vi "Quaternion Between Vectors.vi"(9 "b":dbl[](array[numeric]), 11 "a":dbl[](array[numeric])) -> (3 "quaternion":T1)   [LabVIEW 2013]
uses:
  <vilib>/robotics/Kinematics/Quaternion.ctl
  <vilib>/Analysis/_algsub.llb/Real Vector Norm.vi
  <vilib>/Analysis/baseanly.llb/Real Dot Product.vi
  <vilib>/Analysis/NI_AALPro.lvlib
  <vilib>/Analysis/NI_AALBase.lvlib
  <vilib>/robotics/Kinematics/NI_Kinematics.lvlib
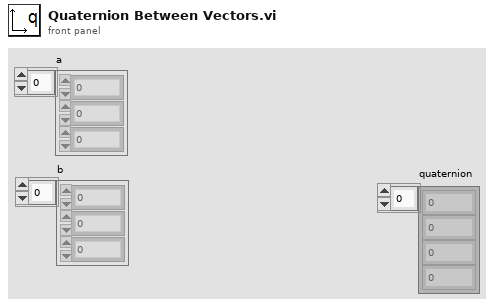
[diagram p1: front panel]
types:
  T1 = typedef "NI_Kinematics.lvlib/Quaternion.ctl" = dbl[]
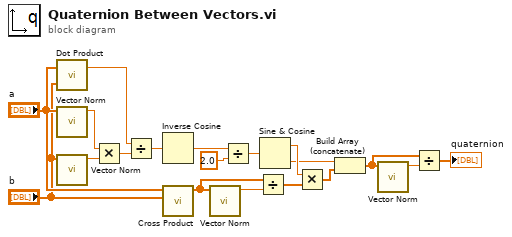
[diagram p0: block diagram]
diagram:
  n1 = call-poly <vilib>:"Dot Product.vi"("Y Vector"="b", "X Vector"="a") -> ("X * Y"=w19:dbl)  [unwired: 1 out]
  n2 = call-poly <vilib>:"Vector Norm.vi"("Input Vector"="a") -> ("norm"=w18:dbl)  [unwired: 9 in, 1 out]
  n3 = call-poly <vilib>:"Vector Norm.vi"("Input Vector"="b") -> ("norm"=w15:dbl)  [unwired: 9 in, 1 out]
  n4 = Multiply(x=w18, y=w15) -> (x*y=w14:dbl)
  n5 = Divide(x=w19, y=w14) -> (x/y=w13:dbl)
  n6 = Inverse Cosine(1:w13) -> (0:w5:dbl)
  n7 = call <vilib>:"Cross Product.vi"("B Vector"="b", "A Vector"="a") -> ("Cross Product"=w12:dbl[])  [unwired: 8 in, 1 out]
  n8 = call-poly <vilib>:"Vector Norm.vi"("Input Vector"=w12) -> ("norm"=w11:dbl)  [unwired: 9 in, 1 out]
  n9 = Divide(x=w5, y=2.0) -> (x/y=w10:dbl)
  n10 = Divide(x=w12, y=w11) -> (x/y=w4:dbl[])
  n11 = Sine & Cosine(0:w10) -> (1:w8:dbl, 2:w7:dbl)
  n12 = Multiply(x=w8, y=w4) -> (x*y=w6:dbl[])
  n13 = Build Array (concatenate)(w7, w6) -> (w3:dbl[])
  n14 = call-poly <vilib>:"Vector Norm.vi"("Input Vector"=w3) -> ("norm"=w2:dbl)  [unwired: 9 in, 1 out]
  n15 = Divide(x=w3, y=w2) -> (x/y=→"quaternion":dbl[])
